vi "State cluster.vi"() -> ()   [LabVIEW 2014]
panel:
  in  "Array":T1(array[cluster]) {"VI  Acq. State" items=["Wait", "Start", "Stop"]; "Delay after" format="%<%H:%M:%S>t"; "Gas selection" items=["N2", "Ar"]; "Delay before" format="%<%H:%M:%S>t"}
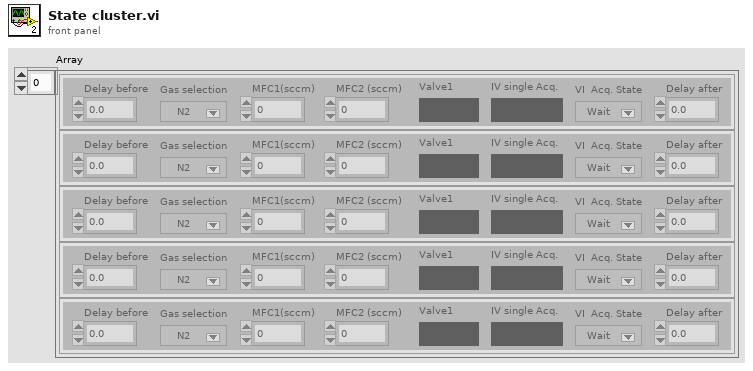
[diagram p1: front panel]
types:
  T1 = cluster{"Delay before":dbl, "Gas selection":u16, "MFC1(sccm) ":dbl, "MFC2 (sccm)":dbl, "Valve1":bool, "Delay after":dbl, "IV single Acq.":bool, "VI  Acq. State":u16}[]
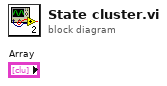
[diagram p0: block diagram]
diagram:
